vi "Convert Command Data 5.0.vi"(11 "Pre 5.0 Command Data":cluster{"Time (s)":dbl, T2, bool}[](array[cluster])) -> (3 "5.0 Command Data":T1)   [LabVIEW 2025]
uses:
  Types/Single Cmd Info.ctl
  <vilib>/picture/picture.llb/imagedata.ctl
  Types/Full Command Info.ctl
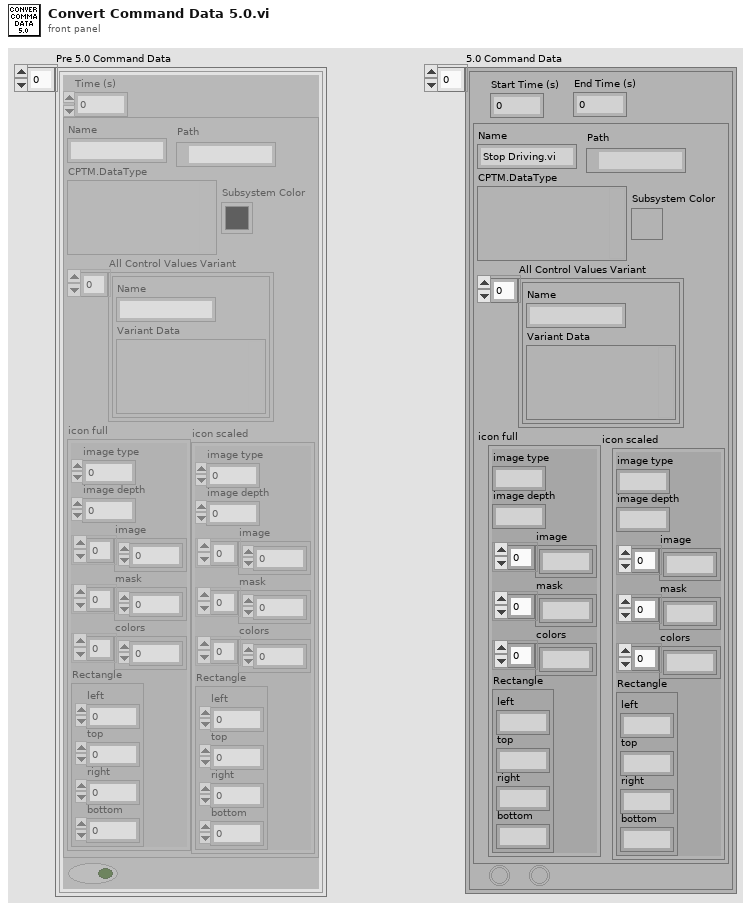
[diagram p1: front panel]
types:
  T1 = typedef "Full Command Info.ctl" = cluster{"Start Time (s)":dbl, "End Time (s)":dbl, T2, "Visible":bool, "Enabled?":bool}[]
  T2 = typedef "Single Cmd Info.ctl" = cluster{"Name":string, "CPTM.DataType":variant, "All Control Values Variant":cluster{"Name":string, "Variant Data":variant}[], "icon full":T3, "icon scaled":T3, "Path":path, "Subsystem Color":u32}
  T3 = typedef "imagedata.ctl" = cluster{"image type":i32, "image depth":i32, "image":u8[], "mask":u8[], "colors":u32[], "Rectangle":cluster{"left":i16, "top":i16, "right":i16, "bottom":i16}}
  T4 = cluster{"Start Time (s)":dbl, "End Time (s)":dbl, T2, "Visible":bool, "Enabled?":bool}
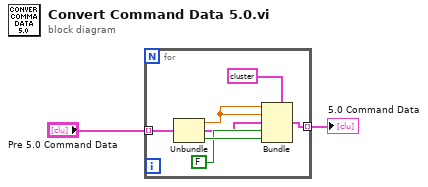
[diagram p0: block diagram]
diagram:
  n1 = for {
    tunnel: "Pre 5.0 Command Data" -> [w9] mode=indexing
    tunnel: [w8] -> w1 mode=indexing
    n2 = Unbundle(w9) -> ("Time (s)"=w7:dbl, w3:T2, w5:bool)
    n3 = Bundle(cluster=T4 data[4986B], "Start Time (s)"=w7, "End Time (s)"=w7, w3, "Visible"=FALSE, "Enabled?"=w5) -> (w8:T4)
  }
  "5.0 Command Data" <- w1
